vi "AttributeToString.vi"   [LabVIEW 2016, in "XML.lvlib" / "XMLAttributeGenerator.lvclass"]
doc: "The polymorphic VI to handle formatting either an array of attributes or a single attribute cluster."
uses:
  <userlib>/Common/XML/XMLAttributeGenerator/XMLAttributeGenerator.lvclass
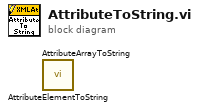
[diagram p0: block diagram]
diagram:
  n1 = call <userlib>:"AttributeElementToString.vi"() -> ()  [unwired: 9 in, 3 out]
  n2 = call <userlib>:"AttributeArrayToString.vi"() -> ()  [unwired: 9 in, 3 out]
